vi "Ratemeter.vi"() -> ()   [LabVIEW 2021]
uses:
  <userlib>/SciSDK/SciSDK_Labview.lvlib
panel:
  out "CH3":dbl
  out "CH2":dbl
  out "CH1":dbl
  out "CH0":dbl
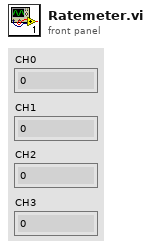
[diagram p1: front panel]
types:
  T1 = cluster{"Name":string, "Board Model":string, "Handle":u64}
  T2 = cluster{"Board Name":string, "Board Model":string, "Handle":u64}
  T3 = cluster{"Ratemeter Path":string, "Ratemeter Name":string}
  T4 = cluster{"magic":u32, "buffer_size":u32, "valid_data":u32, "nchannels":u32, "input":dbl[]}
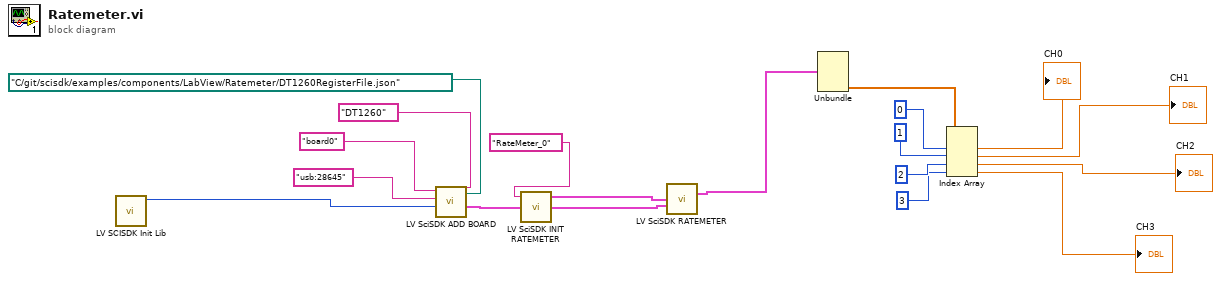
[diagram p0: block diagram]
diagram:
  n1 = call <userlib>:"LV SCISDK Init Lib.vi"() -> ("function return"=w10:u64)  [unwired: 11 in]
  n2 = call <userlib>:"LV SciSDK ADD BOARD.vi"("JsonFile"=path "C:/git/scisdk/examples/components/LabView/Ratemeter/DT1260RegisterFile.json", "Board Model"="DT1260", "SciSDK Handle"=w10, "DevicePath"="usb:28645", "Name"="board0") -> ("Board Handle Out"=w5:T1)  [unwired: 4 in, 2 out]
  n3 = call <userlib>:"LV SciSDK INIT RATEMETER.vi"("Board Handle In"=w5, "Ratemeter Name"="RateMeter_0") -> ("Board Handle Out"=w2:T2, "Digitizer Handle Out"=w3:T3)  [unwired: 1 in, 1 out]
  n4 = call <userlib>:"LV SciSDK RATEMETER.vi"("Ratemeter Handle In"=w3, "Board Handle In"=w2) -> ("Ratemeter Buffer Out"=w1:T4)  [unwired: 9 in, 4 out]
  n5 = Unbundle(w1) -> ("input"=w19:dbl[])  [unwired: 4 out]
  n6 = Index Array(array=w19, index #1=0 ("index"), index #2=1 ("index"), index #3=2 ("index"), index #4=3 ("index")) -> (element #1=→"CH0":dbl, element #2=→"CH1":dbl, element #3=→"CH2":dbl, element #4=→"CH3":dbl)
